vi "ADIS16470 Open.vi"(8 "error in":errorcluster, 10 "Sychronous Process VI":T1, 11 "Hardware Config":T3={"SPI Clock Rate (Hz)"=1000000.0, "IMU SPI Mode (3)"=enum."Mode 3 (Clk Idle High,Sample on Trailing)", "IMU Reset Pin"=enum."SPI Port CS2", "IMU SPI Bus"=enum."SPI On-Board, CS0", "IMU Data Ready Pin"=enum."SPI Port CS1"}) -> (0 "error out":errorcluster, 3 "ADIS16470DevRef":T2={"DevStatus"={"status"=FALSE, "code"=0, "source"=""}, "Hardware Config"={"SPI Clock Rate (Hz)"=1000000.0, "IMU SPI Mode (3)"=enum."Mode 3 (Clk Idle High,Sample on Trailing)", "IMU Reset Pin"=enum."SPI Port CS2", "IMU SPI Bus"=enum."SPI On-Board, CS0", "IMU Data Ready Pin"=enum."SPI Port CS1"}, "End Calibration"=refnum, "Calibration Complete"=refnum, "Data FIFO"=refnum, "Status FIFO"=refnum, "Last Value Reference"=refnum, "Sychronous Process VI"=refnum, "Cmd FIFO"=refnum})   [LabVIEW 2018]
uses:
  Typedef/ADIS16470 Hardware Configuration.ctl
  <vilib>/Rock Robotics/WPI/SPI/WPI_SPIMode.ctl
  <vilib>/Rock Robotics/SystemInterfaces/DIO/FPGA_DIOChannel.ctl
  <vilib>/Rock Robotics/SystemInterfaces/spilib/spi_bus.ctl
  Typedef/ADIS16470 Device Reference.ctl
  Typedef/ADIS16470 Data.ctl
  Typedef/ADIS16470 Status.ctl
  Typedef/ADIS16470 Process.ctl
  Typedef/ADIS16470 Command Type.ctl
  <vilib>/Rock Robotics/SystemInterfaces/NetworkCommunication/NetComm_UsageReport_ResourceType.ctl
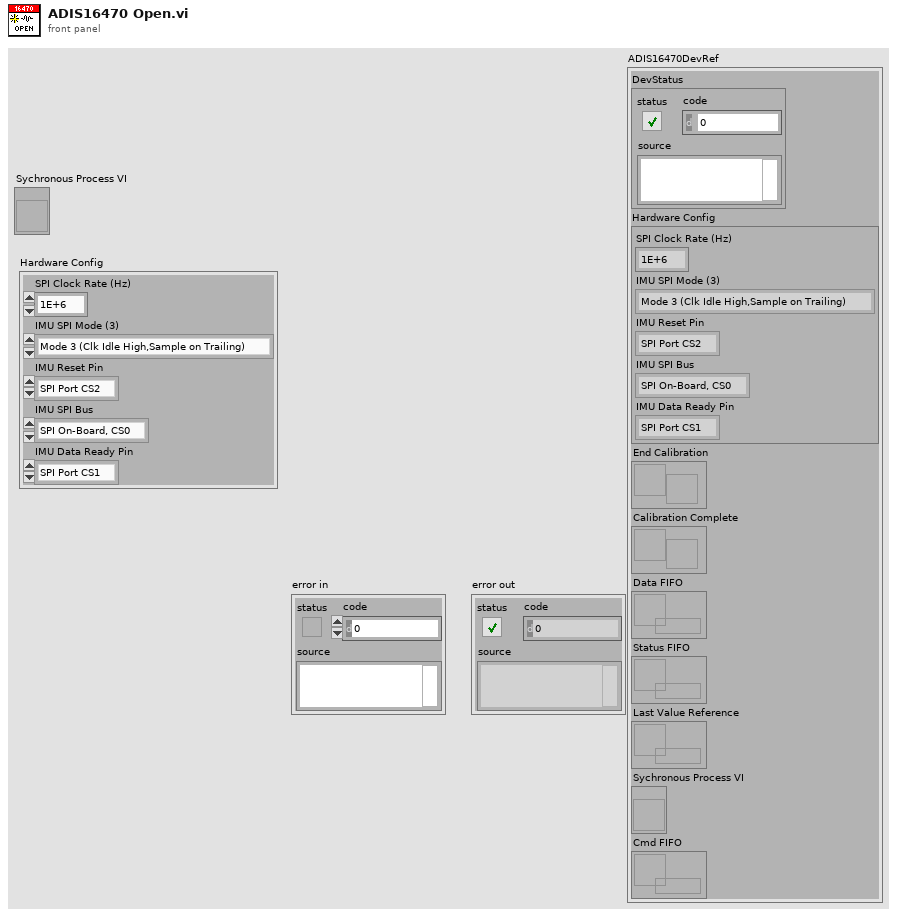
[diagram p1: front panel]
types:
  T1 = typedef "ADIS16470 Process.ctl" = refnum<vi>
  T2 = typedef "ADIS16470 Device Reference.ctl" = cluster{"DevStatus":errorcluster, "Hardware Config":T3, "End Calibration":refnum<notifier>, "Calibration Complete":refnum<notifier>, "Data FIFO":refnum<k33>, "Status FIFO":refnum<k33>, "Last Value Reference":refnum<data-value>, "Sychronous Process VI":T1, "Cmd FIFO":refnum<k33>}
  T3 = typedef "ADIS16470 Hardware Configuration.ctl" = cluster{"SPI Clock Rate (Hz)":dbl, "IMU SPI Mode (3)":T4, "IMU Reset Pin":T5, "IMU SPI Bus":T6, "IMU Data Ready Pin":T5}
  T4 = typedef "WPI_SPIMode.ctl" = enum16{"Mode 0 (Clk Idle Low,Sample on Leading)", "Mode 1 (Clk Idle Low,Sample on Trailing)", "Mode 2 (Clk Idle High,Sample on Leading)", "Mode 3 (Clk Idle High,Sample on Trailing)"}
  T5 = typedef "FPGA_DIOChannel.ctl" = enum8{"DIO 0", "DIO 1", "DIO 2", "DIO 3", "DIO 4", "DIO 5", "DIO 6", "DIO 7", "DIO 8", "DIO 9", "DIO MXP 0", "DIO MXP 1", "DIO MXP 2", "DIO MXP 3", "DIO MXP 4", "DIO MXP 5", "DIO MXP 6", "DIO MXP 7", "DIO MXP 8", "DIO MXP 9", "DIO MXP 10", "DIO MXP 11", "DIO MXP 12", "DIO MXP 13", "DIO MXP 14", "DIO MXP 15", "SPI Port CS1", "SPI Port CS2", "SPI Port CS3", "SPI Port MISO", "SPI Port MOSI", "Invalid"}
  T6 = typedef "spi_bus.ctl" = enum16{"SPI On-Board, CS0", "SPI On-Board, CS1", "SPI On-Board, CS2", "SPI On-Board, CS3", "SPI MXP", "Invalid"}
  T7 = typedef "ADIS16470 Command Type.ctl" = enum16{"None", "Reset"}
  T8 = typedef "ADIS16470 Data.ctl" = cluster{"Yaw":dbl, "Timestamp":dbl, "Timestamp Delta":dbl, "Sample Count":u16}
  T9 = typedef "ADIS16470 Status.ctl" = cluster{"Calibrated?":bool}
  T10 = typedef "NetComm_UsageReport_ResourceType.ctl" = enum8{"Controller", "Module", "Language", "CANPlugin", "Accelerometer", "ADXL345", "AnalogChannel", "AnalogTrigger", "AnalogTriggerOutput", "CANJaguar", "Compressor", "Counter", "Dashboard", "DigitalInput", "DigitalOutput", "DriverStationCIO", "DriverStationEIO", "DriverStationLCD", "Encoder", "GearTooth", "Gyro", "I2C", "Framework", "Jaguar", "Joystick", "Kinect", "KinectStick", "PIDController", "Preferences", "PWM", "Relay", "RobotDrive", "SerialPort", "Servo", "Solenoid", "SPI", "Task", "Ultrasonic", "Victor", "Button", "Command", "AxisCamera", "PCVideoServer", "SmartDashboard", "Talon", "HiTechnicColorSensor", "HiTechnicAccel", "HiTechnicCompass", "SRF08", "AnalogOutput", "Victor SP", "Talon SRX", "CAN Talon SRX", "ADXL362 Accel", "ADXRS450 Gyro", "Rev SPARK", "Mindsensors SD540", "Digital Filter", "ADIS16448", "PDP", "PCM", "PigeonIMU", "Nidec Brushless", "CTRE CANifier", "CTRE Future 0", "CTRE Future 1", "CTRE Future 2", "CTRE Future 3", "CTRE Future 4", "CTRE Future 5", "CTRE Future 6", "Linear Filter", "Xbox Controller", "USB Camera", "NavX", "Pixy", "Pixy2", "ScanseSweep", "Shuffleboard", "CAN", "Digilent DMC60", "PWM Victor SPX", "Rev SPARK MAX PWM", "Rev SPARK MAX CAN", "ADIS16470"}
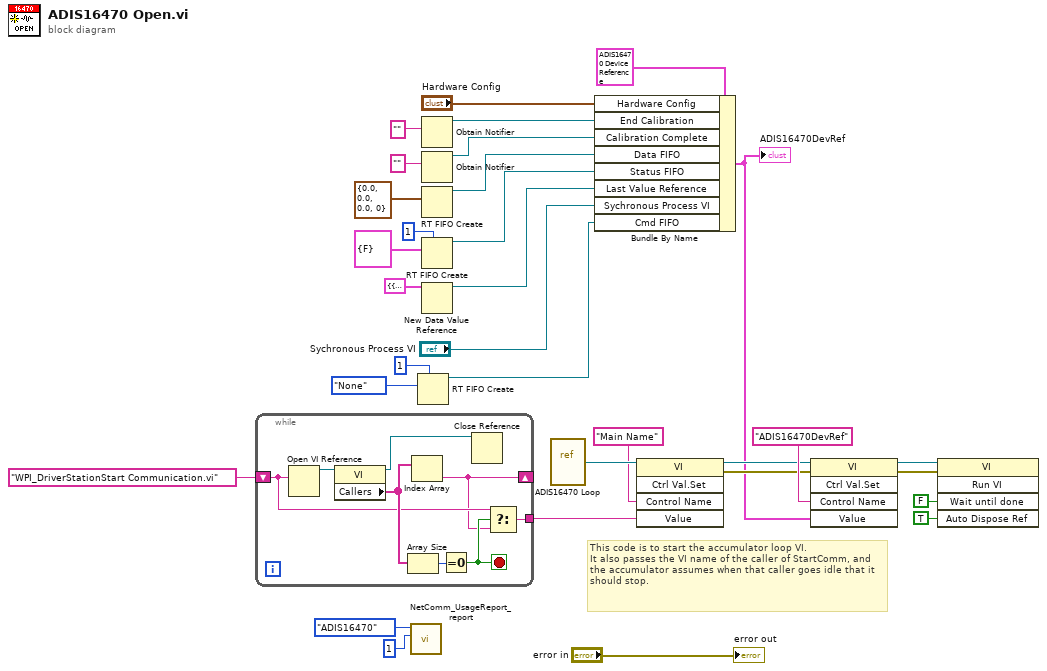
[diagram p0: block diagram]
diagram:
  # "This code is to start the accumulator loop VI.\nIt also passes the VI name of the caller of StartComm, and the accumulator assumes when that caller goes idle that it should stop."
  n1 = while {
    shift-right: [w35] -> _
    shift-left: "WPI_DriverStationStart Communication.vi" -> [w36]
    tunnel: [w34] -> w20
    stop <- w37 stop-if-true
    n2 = Open VI Reference(vi path=w36) -> (vi reference=w40:refnum<vi>)  [unwired: 1 in, 5 out]
    n3 = property class="VI"(reference=w40) -> (reference out=w33:refnum<vi>, "Callers"=w38:string[])  [unwired: 1 in, 1 out]
    n4 = Array Size(array=w38) -> (size(s)=w39:i32)
    n5 = Index Array(array=w38) -> (element=w35:string)  [unwired: 1 in]
    n6 = Equal To 0?(x=w39) -> (x = 0?=w37:bool)
    n7 = Close Reference(reference=w33) -> ()  [unwired: 1 in, 1 out]
    n8 = Select(t=w36, s=w37, f=w35) -> (s? t:f=w34:string)
  }
  n9 = call <vilib>:"NetComm_UsageReport_report.vi"("Instance Number"=u8 1, "Resource Type"=NetComm_UsageReport_ResourceType."ADIS16470") -> ()  [unwired: 10 in]
  n10 = RT FIFO Create(1:ADIS16470_Command_Type."None", 4:u32 1 ("size (10)")) -> (8:w1:refnum<k33>)  [unwired: 6 in, 2 out]
  n11 = Obtain Notifier(notification data type="") -> (notifier out=w14:refnum<notifier>)  [unwired: 3 in, 2 out]
  n12 = Obtain Notifier(notification data type="") -> (notifier out=w15:refnum<notifier>)  [unwired: 3 in, 2 out]
  n13 = RT FIFO Create(1:T8 {"Yaw"=0.0, "Timestamp"=0.0, "Timestamp Delta"=0.0, "Sample Count"=0}) -> (8:w8:refnum<k33>)  [unwired: 7 in, 2 out]
  n14 = RT FIFO Create(1:T9 {"Calibrated?"=FALSE}, 4:u32 1 ("size (10)")) -> (8:w7:refnum<k33>)  [unwired: 6 in, 2 out]
  n15 = New Data Value Reference(data value=cluster{T8, T9} {{"Yaw"=0.0, "Timestamp"=0.0, "Timestamp Delta"=0.0, "Sample Count"=0}, {"Calibrated?"=FALSE}} ("output cluster")) -> (data value reference=w5:refnum<data-value>)  [unwired: 1 in, 1 out]
  n16 = vi-ref "ADIS16470 Loop.vi"() -> (w22:refnum<vi>)
  n17 = Bundle By Name(cluster=T2 {"DevStatus"={"status"=FALSE, "code"=0, "source"=""}, "Hardware Config"={"SPI Clock Rate (Hz)"=1000000.0, "IMU SPI Mode (3)"=enum."Mode 3 (Clk Idle High,Sample on Trailing)", "IMU Reset Pin"=enum."SPI Port CS2", "IMU SPI Bus"=enum."SPI On-Board, CS0", "IMU Data Ready Pin"=enum."SPI Port CS1"}, "End Calibration"=refnum, "Calibration Complete"=refnum, "Data FIFO"=refnum, "Status FIFO"=refnum, "Last Value Reference"=refnum, "Sychronous Process VI"=refnum, "Cmd FIFO"=refnum} ("ADIS16470DevRef"), "Hardware Config"="Hardware Config", "End Calibration"=w14, "Calibration Complete"=w15, "Data FIFO"=w8, "Status FIFO"=w7, "Last Value Reference"=w5, "Sychronous Process VI"="Sychronous Process VI", "Cmd FIFO"=w1) -> (w16:T2)
  "ADIS16470DevRef" <- w16
  n18 = invoke class="VI" method="Ctrl Val.Set"(reference=w22, "Control Name"="Main Name", "Value"=w20) -> (reference out=w19:refnum<vi>, error out=w24:errorcluster)  [unwired: 2 in, 3 out]
  n19 = invoke class="VI" method="Ctrl Val.Set"(reference=w19, error in=w24, "Control Name"="ADIS16470DevRef", "Value"=w16) -> (reference out=w29:refnum<vi>, error out=w25:errorcluster)  [unwired: 1 in, 3 out]
  n20 = invoke class="VI" method="Run VI"(reference=w29, error in=w25, "Wait until done"=FALSE ("Wait Until Done"), "Auto Dispose Ref"=TRUE ("Auto Dispose Reference")) -> ()  [unwired: 1 in, 5 out]
  "error out" <- "error in"
